vi "APC_9056_ClearSoftWarning.vi"(0 "WarningIn":u8[](array[numeric])) -> (1 "WarningOut":u8[](array[numeric]))   [LabVIEW 2020]
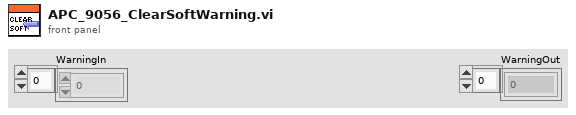
[diagram p1: front panel]
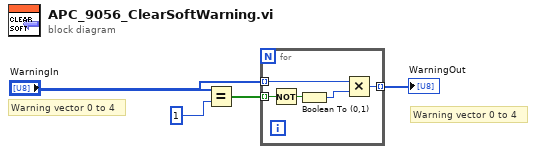
[diagram p0: block diagram]
diagram:
  # "Warning vector 0 to 4"
  # "Warning vector 0 to 4"
  n1 = Equal?(x="WarningIn", y=u8 1 ("lower limit")) -> (x = y?=w3:bool[])
  n2 = for {
    tunnel: w3 -> [w9] mode=indexing
    tunnel: "WarningIn" -> [w6] mode=indexing
    tunnel: [w5] -> w1 mode=indexing
    n3 = Not(x=w9) -> (.not. x?=w8:bool)
    n4 = Boolean To (0,1)(Boolean=w8) -> (0, 1=w7:i16)
    n5 = Multiply(x=w6, y=w7) -> (x*y=w5:i16)
  }
  "WarningOut" <- w1
